vi "Set Currents.vi"() -> (3 "DSM Message":string)   [LabVIEW 2014, in "GEA2_Toolkit.lvlib"]
uses:
  Labview GEA2 Toolkit v2.1/library/GEA2_Toolkit.lvlib
  Custom Pallet Controls/Forward.ctl
panel:
  in  "UE Current (Amps x 10)":u16
  in  "LE Current (Amps x 10)":u16
  in  "Compressor Current (Amps x 10)":u16
  in  "No Load Current (Amps x 10)":u16
  out "Description":string="Set Currents"
  in  "Complete":T1
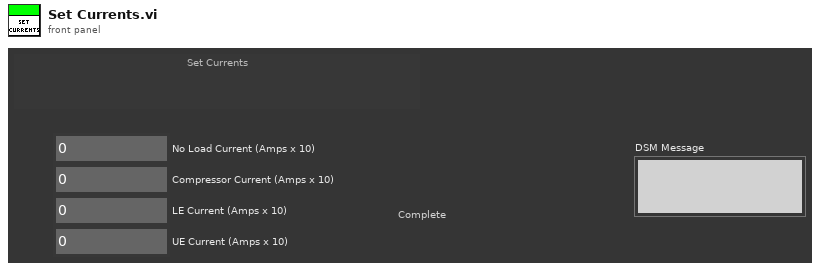
[diagram p1: front panel]
types:
  T1 = typedef "GEA2_Toolkit.lvlib/Forward.ctl" = bool
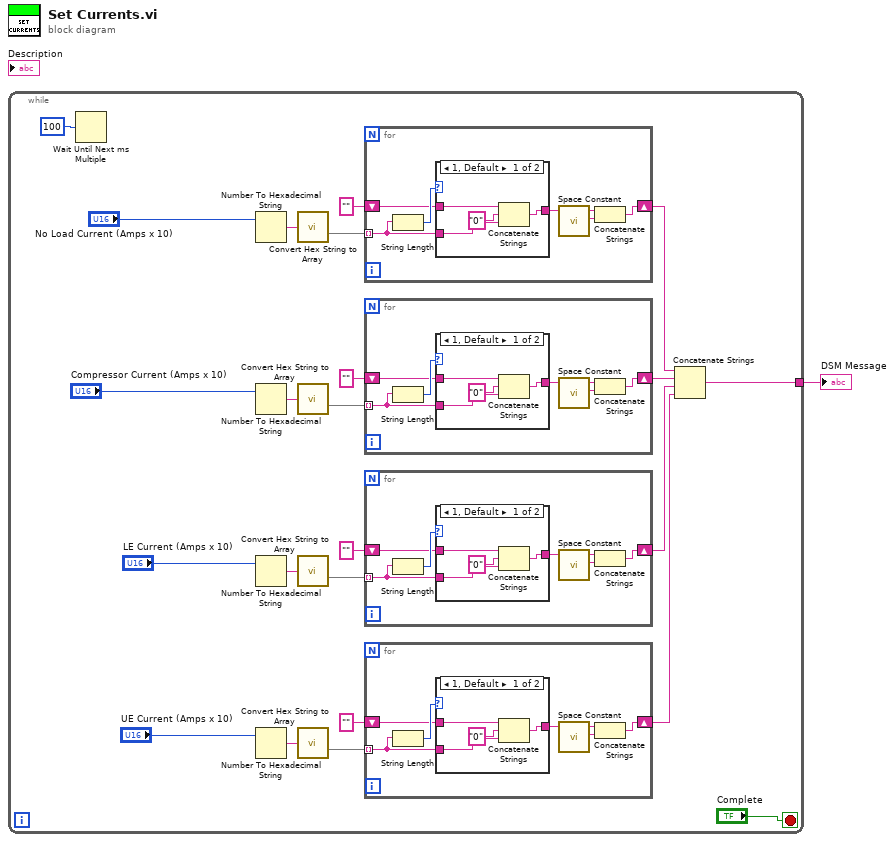
[diagram p0: block diagram]
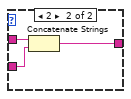
[diagram p2: hidden frame]
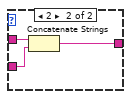
[diagram p3: hidden frame]
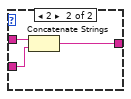
[diagram p4: hidden frame]
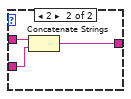
[diagram p5: hidden frame]
diagram:
  n1 = while {
    tunnel: [w5] -> w1
    stop <- "Complete" stop-if-true
    n2 = Wait Until Next ms Multiple(millisecond multiple=u32 100) -> ()  [unwired: 1 out]
    n3 = Number To Hexadecimal String(2:"No Load Current (Amps x 10)") -> (0:w21:string)  [unwired: 1 in]
    n4 = Number To Hexadecimal String(2:"Compressor Current (Amps x 10)") -> (0:w10:string)  [unwired: 1 in]
    n5 = Number To Hexadecimal String(2:"LE Current (Amps x 10)") -> (0:w12:string)  [unwired: 1 in]
    n6 = Number To Hexadecimal String(2:"UE Current (Amps x 10)") -> (0:w14:string)  [unwired: 1 in]
    n7 = call "Convert Hex String to Array.vi"("Hex String In"=w21) -> (10:w20)  [unwired: 13 in, 1 out]
    n8 = call "Convert Hex String to Array.vi"("Hex String In"=w10) -> (10:w18)  [unwired: 13 in, 1 out]
    n9 = call "Convert Hex String to Array.vi"("Hex String In"=w12) -> (10:w17)  [unwired: 13 in, 1 out]
    n10 = call "Convert Hex String to Array.vi"("Hex String In"=w14) -> (10:w16)  [unwired: 13 in, 1 out]
    n11 = for {
      tunnel: w20 -> [w67] mode=indexing
      shift-right: [w64] -> w9
      shift-left: "" -> [w68]
      n12 = String Length(string=w67) -> (length=w69:i32)
      n13 = case shown="1, Default" w69 {
        tunnel: w68 -> [w73 w76]
        tunnel: [w70 w75] -> w65
        tunnel: w67 -> [w71 w74]
        frame 1, Default {
          n14 = Concatenate Strings(w73, "0" ("string"), w71) -> (w70:string)
        }
        frame 2 {
          n15 = Concatenate Strings(w76, w74) -> (w75:string)
        }
      }
      n16 = call <vilib>:"Space Constant.vi"() -> ("String"=w66:string)
      n17 = Concatenate Strings(w65, w66) -> (w64:string)
    }
    n18 = for {
      tunnel: w18 -> [w54] mode=indexing
      shift-right: [w51] -> w8
      shift-left: "" -> [w55]
      n19 = String Length(string=w54) -> (length=w56:i32)
      n20 = case shown="1, Default" w56 {
        tunnel: w55 -> [w60 w63]
        tunnel: [w57 w62] -> w52
        tunnel: w54 -> [w58 w61]
        frame 1, Default {
          n21 = Concatenate Strings(w60, "0" ("string"), w58) -> (w57:string)
        }
        frame 2 {
          n22 = Concatenate Strings(w63, w61) -> (w62:string)
        }
      }
      n23 = call <vilib>:"Space Constant.vi"() -> ("String"=w53:string)
      n24 = Concatenate Strings(w52, w53) -> (w51:string)
    }
    n25 = for {
      tunnel: w17 -> [w41] mode=indexing
      shift-right: [w38] -> w7
      shift-left: "" -> [w42]
      n26 = String Length(string=w41) -> (length=w43:i32)
      n27 = case shown="1, Default" w43 {
        tunnel: w42 -> [w47 w50]
        tunnel: [w44 w49] -> w39
        tunnel: w41 -> [w45 w48]
        frame 1, Default {
          n28 = Concatenate Strings(w47, "0" ("string"), w45) -> (w44:string)
        }
        frame 2 {
          n29 = Concatenate Strings(w50, w48) -> (w49:string)
        }
      }
      n30 = call <vilib>:"Space Constant.vi"() -> ("String"=w40:string)
      n31 = Concatenate Strings(w39, w40) -> (w38:string)
    }
    n32 = for {
      tunnel: w16 -> [w28] mode=indexing
      shift-right: [w25] -> w6
      shift-left: "" -> [w29]
      n33 = String Length(string=w28) -> (length=w30:i32)
      n34 = case shown="1, Default" w30 {
        tunnel: w29 -> [w34 w37]
        tunnel: [w31 w36] -> w26
        tunnel: w28 -> [w32 w35]
        frame 1, Default {
          n35 = Concatenate Strings(w34, "0" ("string"), w32) -> (w31:string)
        }
        frame 2 {
          n36 = Concatenate Strings(w37, w35) -> (w36:string)
        }
      }
      n37 = call <vilib>:"Space Constant.vi"() -> ("String"=w27:string)
      n38 = Concatenate Strings(w26, w27) -> (w25:string)
    }
    n39 = Concatenate Strings(w9, w8, w7, w6) -> (w5:string)
  }
  "DSM Message" <- w1
